vi "Acquire Mouse.vi"   [LabVIEW 2019, in "Acquire Mouse.lvlib"]
doc: "This template is for the Queued Message Handler design pattern.\n\nThe Event Handling Loop generates messages based on user interface actions.\n\nThe Message Handling Loop processes messages generated by the Event Handling Loop, or by other messages. The messages are string values, so new messages can be added easily to the Message Cases case structure in the Message Handling Loop. Each message cluster can also provide an optional value for Message Data, which is a variant that can be converted to whatever message-specific data is required.a"
uses:
  Acquire Mouse.lvlib
  Data.ctl
  Message Queue/State Name.ctl
  <vilib>/Utility/miscctls.llb/LVPositionTypeDef.ctl
  0c61461a-fa07-4497-8c8c-8d3ef654e9c8.vi
  28161244-a5e9-40eb-a1df-742f0088b54a.vi
  d3c4b927-0bb4-4abe-85fe-2b0125df0f06.vi
  681f6a39-68c9-4eb8-ab39-fd2fc03f9966.vi
  <vilib>/Utility/error.llb/Clear Errors.vi
  Message Queue/Enqueue (Single).vi
  <vilib>/Utility/error.llb/Error Cluster From Error Code.vi
  Message Queue/Enqueue (Array).vi
  <vilib>/Utility/inputDevices.llb/mouseAcquire.vi
  Message Queue/Reference Queue.vi
  Message Queue/Message Queue.lvlib
types:
  T1 = typedef "Acquire Mouse.lvlib/State Name.ctl" = enum16{"Initialize", "Re-Initialize", "Initialize Data", "Initialize Panel", "[Event Structure] Update Data", "Add VI", "Get Splitters", "Map Splitter Pos to Coords", "Initialize Mouse", "Acquire Data", "Process Data", "Error", "Exit", "Default"}
  T2 = typedef "Acquire Mouse.lvlib/Data.ctl" = cluster{"Exit":bool, "States":T1, "Mouse ID":refnum<k1>, "Mouse Data":cluster{"axis info":cluster{"Horizontal":i32, "Vertical":i32, "Scrolling":i32}, "Buttons":cluster{"button 1":bool, "button 2":bool, "button 3":bool, "button 4":bool}}, "VIs":refnum<vi>[], "Splitters Info":cluster{"Ref":refnum<vi>, "Name":string, "Owning VI":refnum<vi>, "Position":T3, "IsVertical?":bool, "Position":i32}[]}
  T3 = typedef "LVPositionTypeDef.ctl" = cluster{"Left":i32, "Top":i32}
  T4 = typedef "Message Queue Ref.ctl" = refnum<queue>
  T5 = typedef "Message Queue.lvlib/State Name.ctl" = enum16{"Default", "Initialize", "Initialize Data", "Initialize Modules", "Initialize Panel", "Close FP", "Open FP", "Initialize Menu", "Mode", "Update Subpanel", "Error", "Open Help", "About", "Open WebResources", "Exit"}
  T6 = cluster{refnum<vi>, "Label.Text":string, "VI Refnum":refnum<vi>, "Position":T3, "IsVertical?":bool, "Position":i32}
  T7 = cluster{"Ref":refnum<vi>, "Name":string, "Owning VI":refnum<vi>, "Position":T3, "IsVertical?":bool, "Position":i32}[]
  T8 = typedef "LVRectTypeDef.ctl" = cluster{"Left":i16, "Top":i16, "Right":i16, "Bottom":i16}
  T9 = cluster{"Ref":refnum<vi>, "Name":string, "Owning VI":refnum<vi>, "Position":T3, "IsVertical?":bool, "Position":i32}
  T10 = cluster{"Horizontal":i32, "Vertical":i32, "Scrolling":i32}
  T11 = cluster{"button 1":bool, "button 2":bool, "button 3":bool, "button 4":bool}
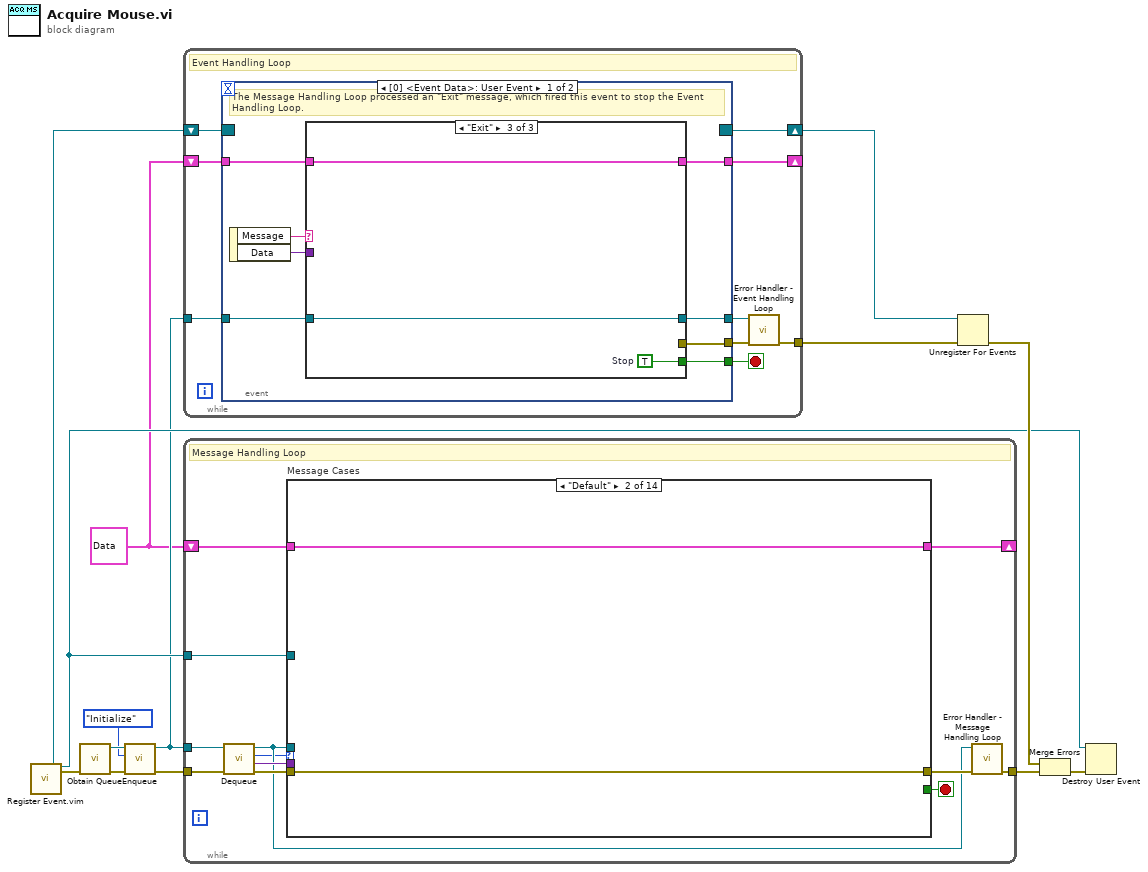
[diagram p0: block diagram]
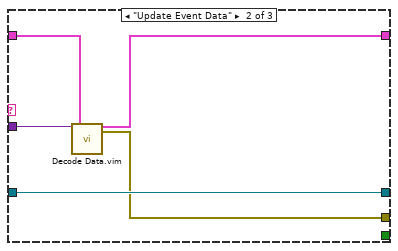
[diagram p3: hidden frame]
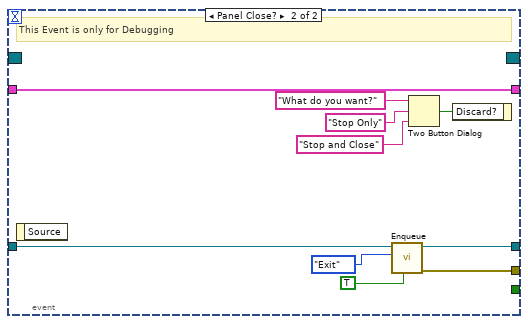
[diagram p4: hidden frame]
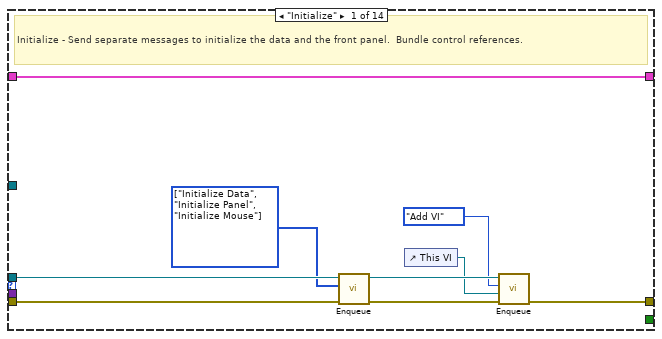
[diagram p5: hidden frame]
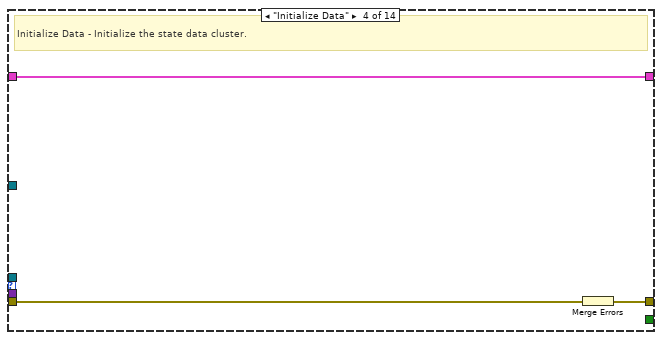
[diagram p7: hidden frame]
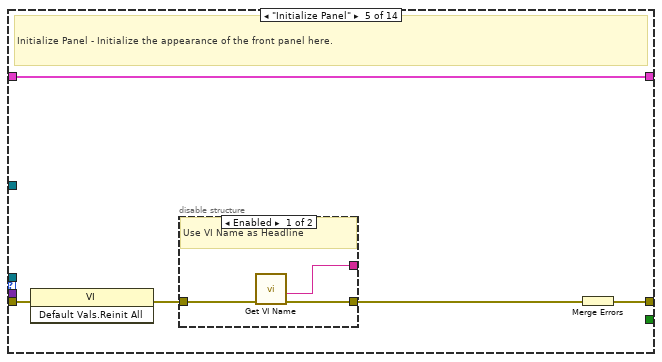
[diagram p8: hidden frame]
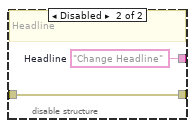
[diagram p9: hidden frame]
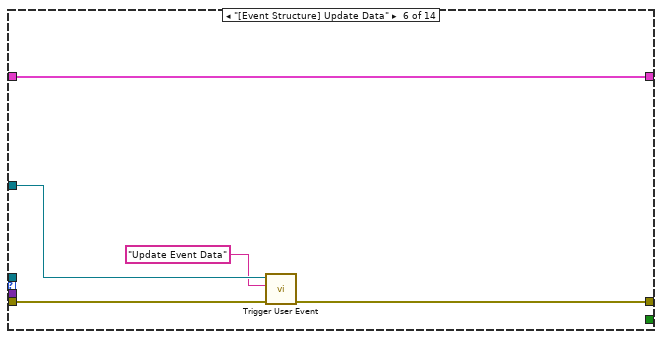
[diagram p10: hidden frame]
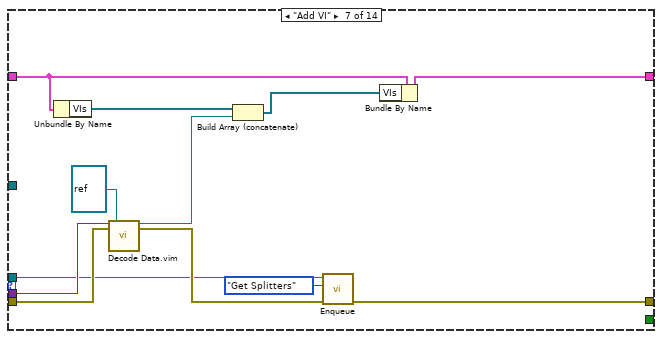
[diagram p11: hidden frame]
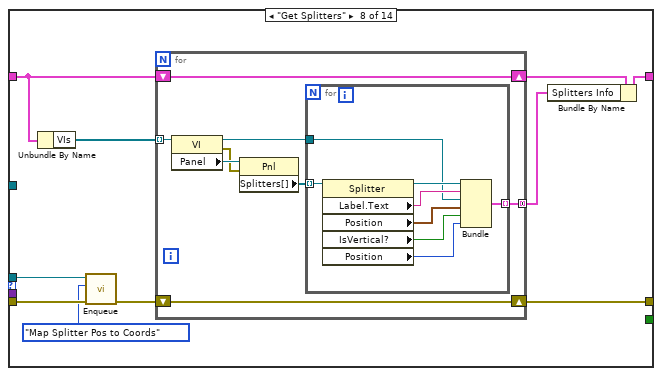
[diagram p12: hidden frame]
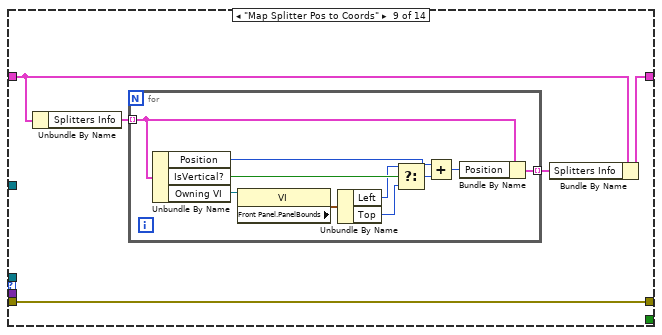
[diagram p13: hidden frame]
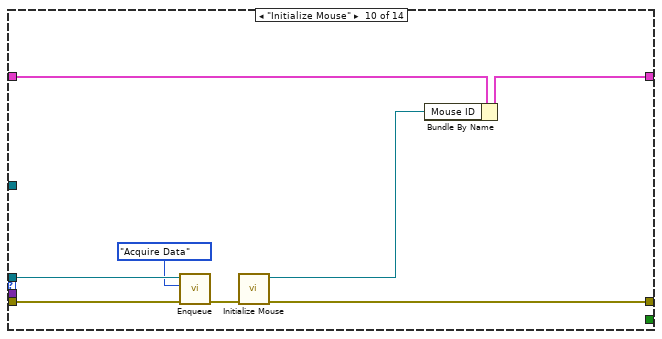
[diagram p14: hidden frame]
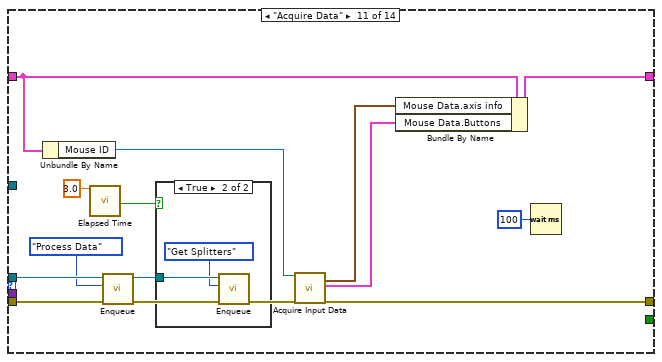
[diagram p15: hidden frame]
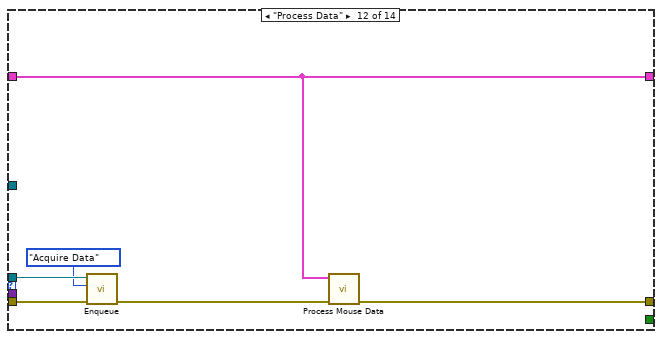
[diagram p17: hidden frame]
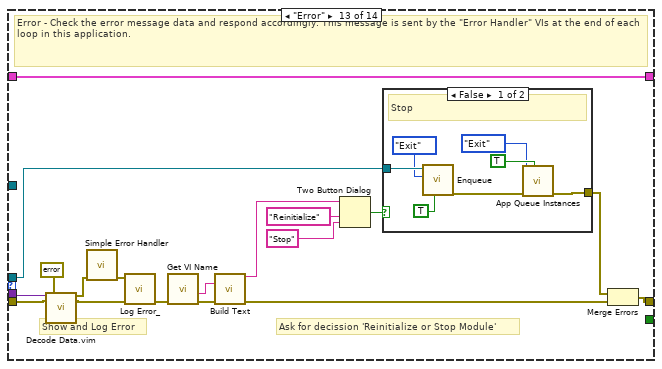
[diagram p18: hidden frame]
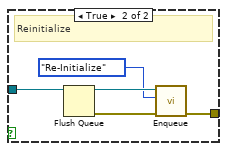
[diagram p19: hidden frame]
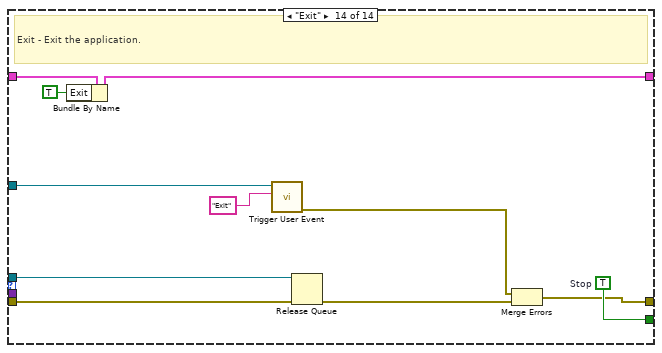
[diagram p20: hidden frame]
diagram:
  w1 = T2 {"Exit"=FALSE, "States"=enum."Initialize", "Mouse ID"=refnum, "Mouse Data"={"axis info"={"Horizontal"=0, "Vertical"=0, "Scrolling"=0}, "Buttons"={"button 1"=FALSE, "button 2"=FALSE, "button 3"=FALSE, "button 4"=FALSE}}, "VIs"=[], "Splitters Info"=[]} ("Data")
  n1 = call "Register Event.vim"() -> ("Registration"=w5:refnum<event-registration>, "user event out"=w4:refnum<user-event>, "error out"=w6:errorcluster)  [unwired: 17 in]
  n2 = call "Obtain Queue.vi"("error in (no error)"=w6) -> ("error out"=w10:errorcluster, "Message Queue"=w11:T4)  [unwired: 9 in]
  n3 = call-poly "Enqueue.vi"("error in (no error)"=w10, "States"=State_Name."Initialize", "Message Queue"=w11) -> ("error out"=w9:errorcluster, "Message Queue dub"=w3:T4)  [unwired: 7 in]
  n4 = while {
    tunnel: w3 -> [w23]
    shift-right: [w15] -> w8
    shift-left: w5 -> [w16]
    tunnel: [w20] -> w12
    shift-right: [w17] -> _
    shift-left: w1 -> [w18]
    stop <- w22 stop-if-true
    # "Event Handling Loop"
    n5 = event shown="[0] <Event Data>: User Event" {
      selector: w16 -> [_ _]
      dyn-events: [_ _] -> w15
      timeout: _ -> [_ _]
      tunnel: [w28 _] -> w22
      tunnel: w23 -> [w31 w44]
      tunnel: [w29 w45] -> w19
      tunnel: [w30 w46] -> w21
      tunnel: w18 -> [w27 w42]
      tunnel: [w24 w42] -> w17
      event User Event {
        # "The Message Handling Loop processed an \"Exit\" message, which fired this event to stop the Event Handling Loop."
        n6 = event-data() -> ("Message"=w25:string, "Data"=w26:variant)  [unwired: 1 in]
        n7 = case shown="\"Exit\"" w25 {
          tunnel: [_ _ w41] -> w28
          tunnel: [_ w34 _] -> w29
          tunnel: w26 -> [_ w38 _]
          tunnel: [w33 w35 w40] -> w30
          tunnel: w31 -> [w33 w35 w40]
          tunnel: [w32 w36 w39] -> w24
          tunnel: w27 -> [w32 w37 w39]
          frame Default {
          }
          frame "Update Event Data" {
            n8 = call "Decode Data.vim"("Data"=w38, "Type/Default value"=w37) -> ("Data out"=w36:T2, "error out"=w34:errorcluster)  [unwired: 16 in]
          }
          frame "Exit" {
            w41 = TRUE  # Stop
          }
        }
      }
      event Panel Close? {
        # "This Event is only for Debugging"
        n9 = event-data() -> ()  [unwired: 1 in, 1 out]
        n10 = call-poly "Enqueue.vi"("Priority Message? Array"=TRUE ("Priority Message? (F)"), "States"=State_Name."Exit" ("Array"), "Message Queue"=w44) -> ("error out"=w45:errorcluster, "Message Queue dub"=w46:T4)  [unwired: 7 in]
        n11 = Two Button Dialog(message="What do you want?", 1:"Stop and Close" ("F button name (\"Cancel\")"), 2:"Stop Only" ("T button name (\"OK\")")) -> (T button?=w48:bool)
        n12 = event-data("Discard?"=w48) -> ()  [unwired: 1 in, 1 out]
      }
    }
    n13 = call "Error Handler - Event Handling Loop.vi"("error in (no error)"=w19, "Message Queue"=w21) -> ("dup error in"=w20:errorcluster)  [unwired: 8 in, 1 out]
  }
  n14 = while {
    tunnel: w3 -> [w58]
    tunnel: w9 -> [w61]
    tunnel: [w57] -> w14
    shift-right: [w53] -> _
    shift-left: w1 -> [w63]
    tunnel: w4 -> [w52]
    stop <- w62 stop-if-true
    # "Message Handling Loop"
    n15 = call "Dequeue.vi"("error in (no error)"=w61, "Message Queue"=w58) -> ("error out"=w60:errorcluster, "Message Data"=w59:variant, "State"=w54:T1, "Message Queue dub"=w55:T4)  [unwired: 4 in, 2 out]
    n16 = case "Message Cases" shown="\"Default\"" w54 {
      tunnel: w55 -> [w71 _ _ _ _ _ w96 w108 _ w149 w161 w175 w184 w218]
      tunnel: w60 -> [w72 w74 w76 w77 w82 w93 w106 w110 w137 w151 w163 w176 w182 w214]
      tunnel: [w68 w74 w76 w79 w84 w92 w97 w116 w137 w154 w168 w172 w183 w215] -> w56
      tunnel: w63 -> [w70 w73 w75 w78 w83 w94 w104 w115 w136 w155 w167 w177 w195 w213]
      tunnel: [_ _ _ _ _ _ _ _ _ _ _ _ _ w217] -> w62
      tunnel: w59 -> [_ _ _ _ _ _ w105 _ _ _ _ _ w181 _]
      tunnel: [w70 w73 w75 w78 w83 w94 w100 w112 w134 w153 w169 w177 w195 w211] -> w53
      tunnel: w52 -> [_ _ _ _ _ w91 _ _ _ _ _ _ _ w209]
      frame "Initialize" {
        w64 = T1[] [enum."Initialize Data", enum."Initialize Panel", enum."Initialize Mouse"] items=["Initialize", "Re-Initialize", "Initialize Data", "Initialize Panel", "[Event Structure] Update Data", "Add VI", "Get Splitters", "Map Splitter Pos to Coords", "Initialize Mouse", "Acquire Data", "Process Data", "Error", "Exit", "Default"] ("Array")
        # "Initialize - Send separate messages to initialize the data and the front panel.  Bundle control references."
        n17 = call-poly "Enqueue.vi"("error in (no error)"=w72, "States"=w64, "Message Queue"=w71) -> ("error out"=w69:errorcluster, "Message Queue dub"=w67:T4)  [unwired: 7 in]
        n18 = control-ref of="This VI"() -> (w65:refnum<vi>)
        n19 = call-poly "Enqueue.vi"("error in (no error)"=w69, "Message Data Array"=w65, "States"=State_Name."Add VI" ("State"), "Message Queue"=w67) -> ("error out"=w68:errorcluster)  [unwired: 6 in, 1 out]
      }
      frame "Default" {
      }
      frame "Re-Initialize" {
      }
      frame "Initialize Data" {
        # "Initialize Data - Initialize the state data cluster."
        n20 = Merge Errors(w77) -> (w79:errorcluster)
      }
      frame "Initialize Panel" {
        # "Initialize Panel - Initialize the appearance of the front panel here."
        n21 = invoke class="VI" method="Default Vals.Reinit All"(error in=w82) -> (error out=w81:errorcluster)  [unwired: 2 in, 2 out]
        n22 = disable-structure shown="Enabled" {
          disable-tunnel: w81 -> [w87 w88]
          disable-tunnel: [w86 w88] -> w80
          disable-tunnel: [w85 w89] -> _
          frame Enabled {
            # "Use VI Name as Headline"
            n23 = call "Get VI Name.vi"("error in (no error)"=w87) -> ("error out"=w86:errorcluster, "VI Name without extension"=w85:string)  [unwired: 8 in, 1 out]
          }
          frame Disabled {
            w89 = "Change Headline"  # Headline
            # "Headline"
          }
        }
        n24 = Merge Errors(w80) -> (w84:errorcluster)
      }
      frame "[Event Structure] Update Data" {
        n25 = call "Trigger User Event.vi"("error in (no error)"=w93, "Message"="Update Event Data", "user event in"=w91) -> ("error out"=w92:errorcluster)  [unwired: 7 in, 1 out]
      }
      frame "Add VI" {
        n26 = Unbundle By Name(w104) -> ("VIs"=w102:refnum<vi>[])
        n27 = call "Decode Data.vim"("Data"=w105, "error in"=w106, "Type/Default value"=refnum<vi> refnum ("VI Refnum")) -> ("Data out"=w101:refnum<vi>, "error out"=w98:errorcluster)  [unwired: 15 in]
        n28 = Build Array (concatenate)(w102, w101) -> (w99:refnum<vi>[])
        n29 = call-poly "Enqueue.vi"("error in (no error)"=w98, "States"=State_Name."Get Splitters", "Message Queue"=w96) -> ("error out"=w97:errorcluster)  [unwired: 7 in, 1 out]
        n30 = Bundle By Name(cluster=w104, "VIs"=w99) -> (w100:T2)
      }
      frame "Get Splitters" {
        n31 = Unbundle By Name(w115) -> ("VIs"=w113:refnum<vi>[])
        n32 = call-poly "Enqueue.vi"("error in (no error)"=w110, "States"=State_Name."Map Splitter Pos to Coords", "Message Queue"=w108) -> ("error out"=w109:errorcluster)  [unwired: 7 in, 1 out]
        n33 = for {
          shift-right: [w124] -> w116
          shift-left: w109 -> [w124]
          shift-right: [w123] -> w114
          shift-left: w115 -> [w123]
          tunnel: w113 -> [w122] mode=indexing
          tunnel: [w117] -> w111 mode=concatenating
          n34 = property class="VI"(reference=w122) -> (reference out=w118:refnum<vi>, error out=w120:errorcluster, "Panel"=w121:refnum<vi>)  [unwired: 1 in]
          n35 = property class="Pnl"(reference=w121, error in=w120) -> ("Splitters[]"=w119:refnum<vi>[])  [unwired: 2 out]
          n36 = for {
            tunnel: w119 -> [w132] mode=indexing
            tunnel: w118 -> [w129]
            tunnel: [w125] -> w117 mode=indexing
            n37 = property class="Splitter"(reference=w132) -> (reference out=w131:refnum<vi>, "Label.Text"=w130:string, "Position"=w128:T3, "IsVertical?"=w127:bool, "Position"=w126:i32)  [unwired: 1 in, 1 out]
            n38 = Bundle(w131, "Label.Text"=w130, "VI Refnum"=w129, "Position"=w128, "IsVertical?"=w127, "Position"=w126) -> (w125:T6)  [unwired: 1 in]
          }
        }
        n39 = Bundle By Name(cluster=w114, "Splitters Info"=w111) -> (w112:T2)
      }
      frame "Map Splitter Pos to Coords" {
        n40 = Unbundle By Name(w136) -> ("Splitters Info"=w135:T7)
        n41 = for {
          tunnel: w135 -> [w141] mode=indexing
          tunnel: [w139] -> w133 mode=indexing
          n42 = Unbundle By Name(w141) -> ("Position"=w142:i32, "IsVertical?"=w146:bool, "Owning VI"=w147:refnum<vi>)
          n43 = property class="VI"(reference=w147) -> ("Front Panel.PanelBounds"=w138:T8)  [unwired: 1 in, 2 out]
          n44 = Unbundle By Name(w138) -> ("Left"=w145:i16, "Top"=w144:i16)
          n45 = Select(t=w145, s=w146, f=w144) -> (s? t:f=w143:i16)
          n46 = Add(x=w142, y=w143) -> (x+y=w140:i32)
          n47 = Bundle By Name(cluster=w141, "Position"=w140) -> (w139:T9)
        }
        n48 = Bundle By Name(cluster=w136, "Splitters Info"=w133) -> (w134:T2)
      }
      frame "Initialize Mouse" {
        n49 = call-poly "Enqueue.vi"("error in (no error)"=w151, "States"=State_Name."Acquire Data", "Message Queue"=w149) -> ("error out"=w150:errorcluster)  [unwired: 7 in, 1 out]
        n50 = call <vilib>:"Initialize Mouse.vi"("error in (no error)"=w150) -> ("error out"=w154:errorcluster, "device ID"=w152:refnum<k1>)  [unwired: 9 in]
        n51 = Bundle By Name(cluster=w155, "Mouse ID"=w152) -> (w153:T2)
      }
      frame "Acquire Data" {
        n52 = Unbundle By Name(w167) -> ("Mouse ID"=w166:refnum<k1>)
        n53 = call "Elapsed Time"("Time Target (s)"=3.0) -> ("Time has Elapsed"=w156:bool)  [unwired: 11 in, 7 out]
        n54 = call-poly "Enqueue.vi"("error in (no error)"=w163, "States"=State_Name."Process Data", "Message Queue"=w161) -> ("error out"=w162:errorcluster, "Message Queue dub"=w158:T4)  [unwired: 7 in]
        n55 = case shown="True" w156 {
          tunnel: w158 -> [_ w171]
          frame False {
          }
          frame True {
            n56 = call-poly "Enqueue.vi"("States"=State_Name."Get Splitters", "Message Queue"=w171) -> ()  [unwired: 8 in, 2 out]
          }
        }
        n57 = call-poly <vilib>:"Acquire Input Data.vi"("device ID"=w166, "error in (no error)"=w162) -> ("axis info"=w165:T10, "button info"=w164:T11, "error out"=w168:errorcluster)  [unwired: 14 in, 1 out]
        n58 = Bundle By Name(cluster=w167, "Mouse Data.axis info"=w165, "Mouse Data.Buttons"=w164) -> (w169:T2)
        n59 = Wait (ms)(milliseconds to wait=u32 100) -> ()  [unwired: 1 out]
      }
      frame "Process Data" {
        n60 = call-poly "Enqueue.vi"("error in (no error)"=w176, "States"=State_Name."Acquire Data", "Message Queue"=w175) -> ("error out"=w173:errorcluster)  [unwired: 7 in, 1 out]
        n61 = call "Process Mouse Data.vi"("error in"=w173, "Data"=w177) -> ("error out"=w172:errorcluster)  [unwired: 9 in]
      }
      frame "Error" {
        # "Ask for decission 'Reinitialize or Stop Module'"
        # "Show and Log Error"
        # "Error - Check the error message data and respond accordingly. This message is sent by the \"Error Handler\" VIs at the end of each loop in this application."
        n62 = call "Decode Data.vim"("Data"=w181, "error in"=w182, "Type/Default value"=errorcluster {"status"=FALSE, "code"=0, "source"=""} ("error constant")) -> ("Data out"=w178:errorcluster, "error out"=w179:errorcluster)  [unwired: 15 in]
        n63 = call <vilib>:"Simple Error Handler.vi"("error in (no error)"=w178) -> ("error out"=w194:errorcluster)  [unwired: 4 in, 4 out]
        n64 = call "Log Error_.vi"("error in"=w179, "Error log to file"=w194) -> ("error out"=w193:errorcluster)  [unwired: 9 in]
        n65 = call "Get VI Name.vi"("error in (no error)"=w193) -> ("error out"=w189:errorcluster, "VI Name without extension"=w190:string)  [unwired: 8 in, 1 out]
        n66 = call "Build Text"("ModuleName"=w190, "error in (no error)"=w189) -> ("Result"=w192:string, "error out"=w191:errorcluster)  [unwired: 12 in]
        n67 = Two Button Dialog(message=w192, 1:"Stop" ("F button name (\"Cancel\")"), 2:"Reinitialize" ("T button name (\"OK\")")) -> (T button?=w188:bool)
        n68 = case shown="False" w188 {
          tunnel: w184 -> [w202 w207]
          tunnel: [w200 w204] -> w187
          frame False {
            # "Stop"
            n69 = call-poly "Enqueue.vi"("Priority Message? Array"=TRUE ("Priority Message? (F)"), "States"=State_Name."Exit" ("Array"), "Message Queue"=w202) -> ("error out"=w198:errorcluster)  [unwired: 7 in, 1 out]
            n70 = call-poly "App Queue Instances.vi"("Priority Message? (F)"=TRUE, "error in (no error)"=w198, "Tasks"=State_Name."Exit") -> ("error out"=w200:errorcluster)  [unwired: 8 in]
          }
          frame True {
            # "Reinitialize"
            n71 = Flush Queue(queue=w207) -> (queue out=w206:T4, error out=w205:errorcluster)  [unwired: 1 in, 1 out]
            n72 = call-poly "Enqueue.vi"("error in (no error)"=w205, "States"=State_Name."Re-Initialize" ("Array"), "Message Queue"=w206) -> ("error out"=w204:errorcluster)  [unwired: 7 in, 1 out]
          }
        }
        n73 = Merge Errors(w187, w191) -> (w183:errorcluster)
      }
      frame "Exit" {
        w217 = TRUE  # Stop
        # "Exit - Exit the application."
        n74 = Bundle By Name(cluster=w213, "Exit"=TRUE) -> (w211:T2)
        n75 = call "Trigger User Event.vi"("Message"="Exit", "user event in"=w209) -> ("error out"=w210:errorcluster)  [unwired: 8 in, 1 out]
        n76 = Release Queue(queue=w218, error in (no error)=w214) -> (error out=w216:errorcluster)  [unwired: 1 in, 2 out]
        n77 = Merge Errors(w210, w216) -> (w215:errorcluster)
      }
    }
    n78 = call "Error Handler - Message Handling Loop.vi"("error in (no error)"=w56, "Message Queue"=w55) -> ("dup error in"=w57:errorcluster)  [unwired: 8 in, 1 out]
  }
  n79 = Unregister For Events(event registration refnum=w8, error in=w12) -> (error out=w13:errorcluster)
  n80 = Merge Errors(w13, w14) -> (w7:errorcluster)
  n81 = Destroy User Event(user event=w4, error in=w7) -> ()  [unwired: 1 out]
